vi "move fake image.vi"(9 "fake image location":T2) -> (1 "fake image location out":T2, 2 "center location":T1)   [LabVIEW 2010]
uses:
  moving fake image params.ctl
  <vilib>/rvi/FXPMathLib/FxpAdd/XNode/nifxpmath_Add.xnode
  <vilib>/rvi/FXPMathLib/FxpAdd/subVIs/nifxpmath_Add_SimConfig.ctl
  <vilib>/fxp/LVFixedPointQuantizationPolicyTypeDef.ctl
  <vilib>/fxp/LVFixedPointOverflowPolicyTypeDef.ctl
  <vilib>/rvi/FXPMathLib/FxpAdd/simVIs/DllFxpAddTemp_sub.vi
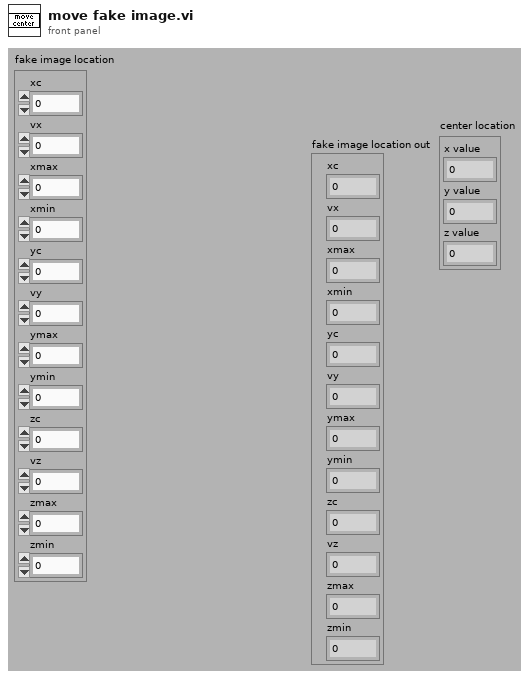
[diagram p1: front panel]
types:
  T1 = cluster{"x value":i16, "y value":i16, "z value":i16}
  T2 = typedef "moving fake image params.ctl" = cluster{"xc":fxp<+/-,32,16>, "vx":fxp<+/-,12,-4>, "xmax":fxp<+/-,32,16>, "xmin":fxp<+/-,32,16>, "yc":fxp<+/-,32,16>, "vy":fxp<+/-,12,-4>, "ymax":fxp<+/-,32,16>, "ymin":fxp<+/-,32,16>, "zc":fxp<+/-,32,16>, "vz":fxp<+/-,12,-4>, "zmax":fxp<+/-,32,16>, "zmin":fxp<+/-,32,16>}
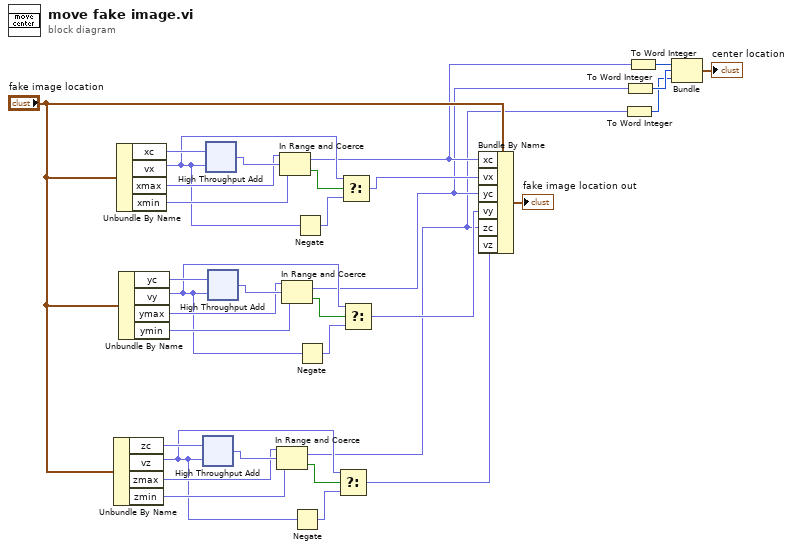
[diagram p0: block diagram]
diagram:
  n1 = Unbundle By Name("fake image location") -> ("zc"=w18:fxp<+/-,32,16>, "vz"=w13:fxp<+/-,12,-4>, "zmax"=w16:fxp<+/-,32,16>, "zmin"=w15:fxp<+/-,32,16>)
  n2 = Unbundle By Name("fake image location") -> ("xc"=w33:fxp<+/-,32,16>, "vx"=w28:fxp<+/-,12,-4>, "xmax"=w31:fxp<+/-,32,16>, "xmin"=w30:fxp<+/-,32,16>)
  n3 = Unbundle By Name("fake image location") -> ("yc"=w25:fxp<+/-,32,16>, "vy"=w20:fxp<+/-,12,-4>, "ymax"=w23:fxp<+/-,32,16>, "ymin"=w22:fxp<+/-,32,16>)
  n4 = xnode "High Throughput Add"("x"=w18, "y"=w13) -> ("x+y"=w17:fxp<+/-,32,16>)
  n5 = xnode "High Throughput Add"("x"=w33, "y"=w28) -> ("x+y"=w32:fxp<+/-,32,16>)
  n6 = xnode "High Throughput Add"("x"=w25, "y"=w20) -> ("x+y"=w24:fxp<+/-,32,16>)
  n7 = In Range and Coerce(upper limit=w16, x=w17, lower limit=w15) -> (coerced(x)=w5:fxp<+/-,32,16>, In Range?=w14:bool)
  n8 = In Range and Coerce(upper limit=w31, x=w32, lower limit=w30) -> (coerced(x)=w7:fxp<+/-,32,16>, In Range?=w29:bool)
  n9 = In Range and Coerce(upper limit=w23, x=w24, lower limit=w22) -> (coerced(x)=w6:fxp<+/-,32,16>, In Range?=w21:bool)
  n10 = Negate(x=w13) -> (-x=w12:fxp<+/-,12,-4>)
  n11 = Negate(x=w28) -> (-x=w27:fxp<+/-,12,-4>)
  n12 = Negate(x=w20) -> (-x=w19:fxp<+/-,12,-4>)
  n13 = Select(t=w13, s=w14, f=w12) -> (s? t:f=w10:fxp<+/-,12,-4>)
  n14 = Select(t=w28, s=w29, f=w27) -> (s? t:f=w26:fxp<+/-,12,-4>)
  n15 = Select(t=w20, s=w21, f=w19) -> (s? t:f=w11:fxp<+/-,12,-4>)
  n16 = Bundle By Name(cluster="fake image location", "xc"=w7, "vx"=w26, "yc"=w6, "vy"=w11, "zc"=w5, "vz"=w10) -> (→"fake image location out":T2)
  n17 = To Word Integer(number=w5) -> (16bit integer=w2:i16)
  n18 = To Word Integer(number=w6) -> (16bit integer=w3:i16)
  n19 = To Word Integer(number=w7) -> (16bit integer=w4:i16)
  n20 = Bundle(w4, w3, w2) -> (→"center location":cluster{i16, i16, i16})  [unwired: 1 in]
